vi "Populate Ctrl.vi"(8 "error in (no error)":errorcluster, 11 "FK Ring in":refnum<class "FK Ring.lvclass">) -> (0 "error out":errorcluster, 3 "FK Ring out":refnum<class "FK Ring.lvclass">)   [LabVIEW 2020, in "Basic Fields.lvlib" / "FK Ring.lvclass"]
uses:
  FK Ring.lvclass
  Column Interface/Column Configuration Interface Class/Column Configuration.lvclass
  Database Libraries/Database Interfaces/Database Interface Class/Database Interface.lvclass
  Basic Fields.lvlib
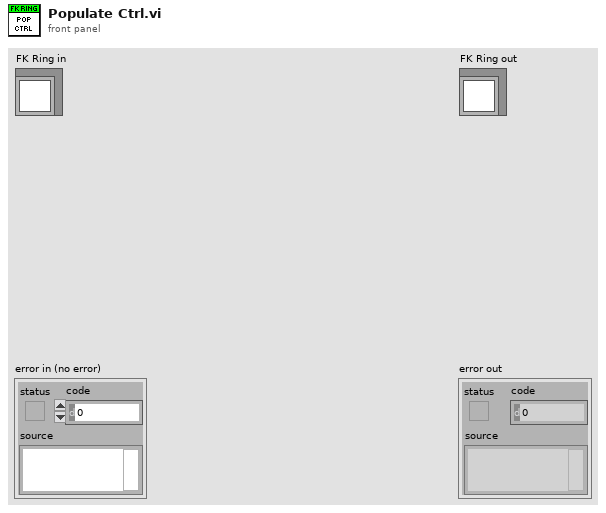
[diagram p1: front panel]
types:
  T1 = typedef "Column Interfaces.lvlib/FK Info.ctl" = cluster{"PK Table":string, "PK Column":string, "PK Display Column":string}
  T2 = typedef "LVStringsAndValuesArrayTypeDef.ctl" = cluster{"String":string, "Value":ext}[]
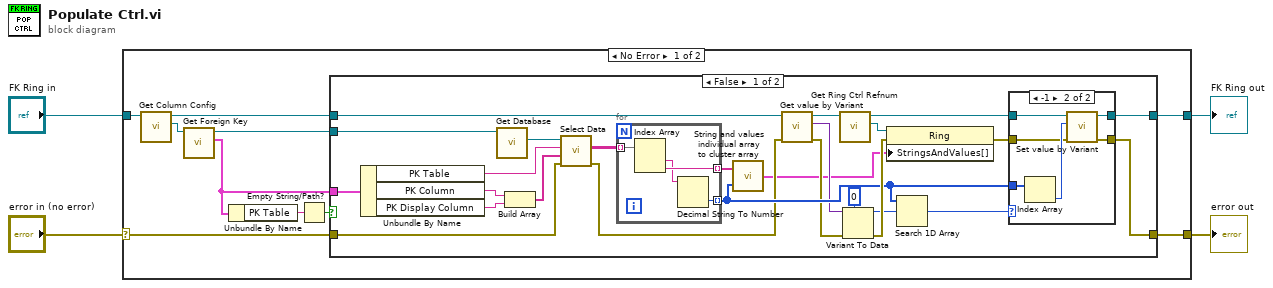
[diagram p0: block diagram]
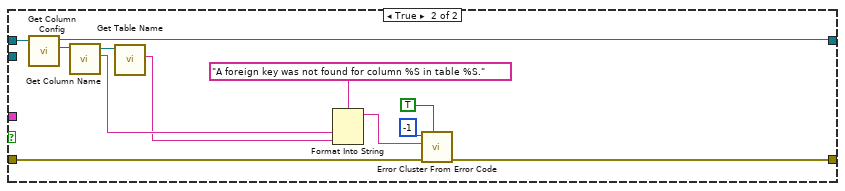
[diagram p3: hidden frame]
diagram:
  n1 = case shown="No Error" "error in (no error)" {
    selector: "error in (no error)" -> [w11 w65]
    tunnel: [w10 w65] -> w3
    tunnel: "FK Ring in" -> [w14 w66]
    tunnel: [w8 w66] -> w1
    frame No Error {
      n2 = call-dynamic "Get Column Config.vi"("Ctrl Refnum Column in"=w14) -> ("Column Configuration"=w13:refnum<class "Column Configuration.lvclass">, "Ctrl Refnum Column out"=w9:refnum<class "FK Ring.lvclass">)  [unwired: 8 in, 1 out]
      n3 = call-dynamic "Get Foreign Key.vi"("Column Configuration in"=w13) -> ("FK Info"=w7:T1, "Column Configuration out"=w12:refnum<class "Column Configuration.lvclass">)  [unwired: 8 in, 1 out]
      n4 = Unbundle By Name(w7) -> ("PK Table"=w6:string)
      n5 = Empty String/Path?(string/path=w6) -> (empty?=w5:bool)
      n6 = case shown="False" w5 {
        tunnel: w12 -> [w40 _]
        tunnel: w11 -> [w34 w54]
        tunnel: [w25 w53] -> w10
        tunnel: w9 -> [w23 w64]
        tunnel: [w16 w60] -> w8
        tunnel: w7 -> [w15 _]
        frame False {
          n7 = Unbundle By Name(w15) -> ("PK Table"=w36:string, "PK Column"=w38:string, "PK Display Column"=w37:string)
          n8 = call-dynamic "Get Database.vi"("Column Configuration in"=w40) -> ("Database"=w39:refnum<class "Database Interface.lvclass">)  [unwired: 8 in, 2 out]
          n9 = Build Array(w38, w37) -> (w35:string[])
          n10 = call-dynamic "Select Data.vi"("error in (no error)"=w34, "Columns"=w35, "Table"=w36, "Database Interface in"=w39) -> ("error out"=w21:errorcluster, "Data"=w33:string[][])  [unwired: 5 in, 1 out]
          n11 = for {
            tunnel: w33 -> [w52] mode=indexing
            tunnel: [w51] -> w32 mode=indexing
            tunnel: [w49] -> w27 mode=indexing
            n12 = Index Array(array=w52) -> (element #1=w50:string, element #2=w51:string)  [unwired: 2 in]
            n13 = Decimal String To Number(string=w50) -> (number=w49:i32)  [unwired: 2 in, 1 out]
          }
          n14 = call "String and values individual array to cluster array.vi"("Value Array In"=w27, "String Array In"=w32) -> ("Strings and Values Out"=w18:T2)
          n15 = call-dynamic "Get value by Variant.vi"("error in (no error)"=w21, "Ctrl Refnum Column in"=w23) -> ("error out"=w20:errorcluster, "Variant"=w19:variant, "Ctrl Refnum Column out"=w22:refnum<class "FK Ring.lvclass">)  [unwired: 7 in]
          n16 = call "Get Ring Ctrl Refnum.vi"("FK Ring in"=w22) -> ("Ring Refnum"=w24:refnum<vi>, "FK Ring out"=w17:refnum<class "FK Ring.lvclass">)  [unwired: 8 in, 1 out]
          n17 = Variant To Data(error in=w20, type=0, Variant=w19) -> (data=w29:i32, error out=w30:errorcluster)
          n18 = property class="Ring"(reference=w24, error in=w30, "StringsAndValues[]"=w18) -> (error out=w26:errorcluster)  [unwired: 1 out]
          n19 = Search 1D Array(1D array=w27, element=w29) -> (index of element=w28:i32)  [unwired: 1 in]
          n20 = case shown="-1" w28 {
            tunnel: w27 -> [_ w48]
            tunnel: w26 -> [w42 w44]
            tunnel: [w42 w43] -> w25
            tunnel: w17 -> [w41 w47]
            tunnel: [w41 w46] -> w16
            frame 0, Default {
            }
            frame -1 {
              n21 = Index Array(array=w48) -> (element=w45:i32)  [unwired: 1 in]
              n22 = call-dynamic "Set value by Variant.vi"("error in (no error)"=w44, "Variant"=w45, "Column in"=w47) -> ("error out"=w43:errorcluster, "Column out"=w46:refnum<class "FK Ring.lvclass">)  [unwired: 7 in]
            }
          }
        }
        frame True {
          n23 = call-dynamic "Get Column Config.vi"("Ctrl Refnum Column in"=w64) -> ("Column Configuration"=w63:refnum<class "Column Configuration.lvclass">, "Ctrl Refnum Column out"=w60:refnum<class "FK Ring.lvclass">)  [unwired: 8 in, 1 out]
          n24 = call-dynamic "Get Column Name.vi"("Column Configuration in"=w63) -> ("Column Name"=w59:string, "Column Configuration out"=w61:refnum<class "Column Configuration.lvclass">)  [unwired: 8 in, 1 out]
          n25 = call-dynamic "Get Table Name.vi"("Column Configuration in"=w61) -> ("Table Name"=w58:string)  [unwired: 8 in, 2 out]
          n26 = Format Into String(format string="A foreign key was not found for column %S in table %S.", w59, w58) -> (resulting string=w57:string)  [unwired: 2 in, 1 out]
          n27 = call <vilib>:"Error Cluster From Error Code.vi"("show call chain? (False)"=TRUE, "error in (no error)"=w54, "error message (\"\")"=w57, "error code (0)"=-1) -> ("error out"=w53:errorcluster)  [unwired: 5 in]
        }
      }
    }
    frame Error {
    }
  }
  "error out" <- w3
  "FK Ring out" <- w1
